vi "Ejercicio_03.vi"() -> ()   [LabVIEW 2020]
panel:
  in  "stop":bool
  out "Tabla Indicador":string[][](table)
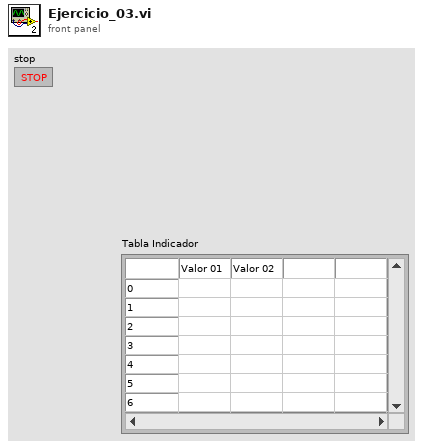
[diagram p1: front panel]
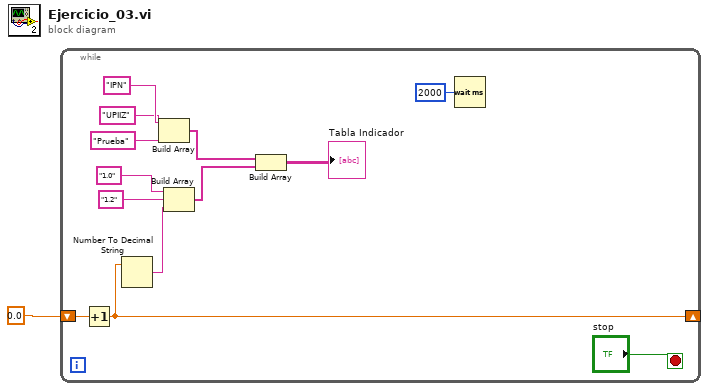
[diagram p0: block diagram]
diagram:
  n1 = while {
    shift-right: [w2] -> _
    shift-left: 0.0 -> [w3]
    stop <- "stop" stop-if-true
    n2 = Increment(x=w3) -> (x+1=w2:dbl)
    n3 = Number To Decimal String(number=w2) -> (decimal integer string=w4:string)  [unwired: 1 in]
    n4 = Build Array("IPN", "UPIIZ", "Prueba") -> (w13:string[])
    n5 = Build Array("1.0", "1.2", w4) -> (w12:string[])
    n6 = Build Array(w13, w12) -> (→"Tabla Indicador":string[][])
    n7 = Wait (ms)(milliseconds to wait=u32 2000) -> ()  [unwired: 1 out]
  }
